vi "Create a Filter Bank from a Prototype Filter.vi"() -> ()   [LabVIEW 2023]
doc: "This example demonstrates how to use the <b>DFD Build Filter Bank from Prototype Filter</b> VI to create a cosine-modulated filter bank from prototype filter coefficients.\n\nComplete the following steps to use this VI:\n1) Run this VI.\n2) On the <b>Frequency Responses</b> tab, observe the magnitude and phase responses of the filter bank.\n3) On the <b>Distortions</b> tab, observe the aliasing, magnitude distortion, and phase distortion in the filter bank. The distortions are small.\n4) Change the value of <b>Band Counts</b>. \n5) Run this VI. Observe the <b>Distortions</b> tab. The distortions are large, which means this filter bank does not have perfect reconstruction. If you change <b>Band Counts</b>, you also must change the <b>Prototype Filter Coefficients</b>.\n6) To design a prototype filter, copy the coefficients to <b>Prototype Filter Coefficients</b> and set the proper value of <b>Band Counts</b>. Observe the frequency responses and distortions."
uses:
  <vilib>/addons/Digital Filter Design/_Objects.llb/DFD Phase Setting.ctl
  <vilib>/addons/Digital Filter Design/FilterBank.llb/FilterBankLib/DFD Build Filter Bank from Filter Coefficients.vi
  <vilib>/addons/Digital Filter Design/NI_DigFilter_FilterBank.lvlib
  <vilib>/addons/Digital Filter Design/NI_DigFilterLicensed.lvlib
panel:
  in  "Tab Control":enum32{"Frequency Responses", "Distortions"}(tab)
  out "Magnitude Responses":cluster{"Y":dbl[], "Y":dbl[]}[](graph)
  out "Phase Responses":cluster{"Y":dbl[], "Y":dbl[]}[](graph)
  out "Aliasing":cluster{dbl[], "values":dbl[]}(graph)
  out "Magnitude Distortion":cluster{dbl[], "values":dbl[]}(graph)
  out "Phase Distortion":cluster{dbl[], "values":dbl[]}(graph)
  in  "Band Counts":i32=4
  in  "Prototype Filter Coefficients":dbl[](array[numeric])=[3.82246474069644e-05, -0.0013784809253753554, 0.009144604896938757, 0.0003140814295197787, 0.00013518515431935828, 0.0003333316277785628, 0.0022112645736163537, -0.001110779285062549, -0.004449412805990734, -0.025388145079228278, -0.023860529399402756, -0.02350561463356747, -0.013170266328729315, 0.012862434811574027, 0.03883151987903549, 0.062049771616075604, 0.08864889782622157, 0.11056100576702955, 0.12668278199988298, 0.1370915002247963, 0.1370915002247963, 0.12668278199988298, 0.11056100576702955, 0.08864889782622157, 0.062049771616075604, 0.03883151987903549, 0.012862434811574027, -0.013170266328729315, -0.02350561463356747, -0.023860529399402756, -0.025388145079228278, -0.004449412805990734, -0.001110779285062549, 0.0022112645736163537, 0.0003333316277785628, 0.00013518515431935828, 0.0003140814295197787, 0.009144604896938757, -0.0013784809253753554, 3.82246474069644e-05]
  # "Select Help>>Show Context Help and move the cursor over the VI icon for more information."
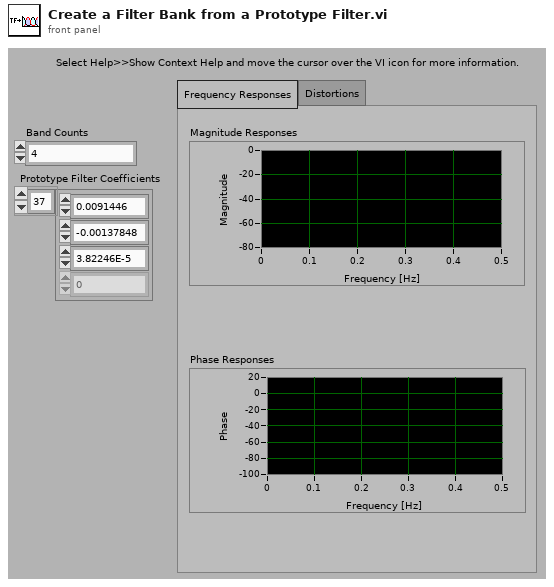
[diagram p1: front panel]
types:
  T1 = typedef "NI_DigFilterLicensed.lvlib/DFD Phase Setting.ctl" = cluster{"unwrap? (F)":bool, "degree? (F)":bool}
  T2 = typedef "NI_DigFilter_FilterBank.lvlib/DFD Filter Bank Obj.ctl" = cluster{"mFBank_AnalysisFilters":T3[], "mFBank_SynthesisFilters":T3[], "mFBank_#Bands":i32, "mFBank_ProcMethod":T8, "mFBank_Coeffs":dbl[], "mFBank_Gain":dbl, "mFBank_Delay":i32, "mFBank_Type":T9}
  T3 = typedef "NI_DigFilterLicensed.lvlib/DFD Multirate Filter Obj.ctl" = cluster{"mMRate_Structure":enum16{"CIC", "FIR", "IIR", "Lattice"}, "mMRate_Mode":T4, "mMRate_Factor":i32, "mMRate_FIRParams":cluster{"mMRate_FIR_H":dbl[], "mMRate_FIR_IsNyquist?":bool, "mMRate_FIR_IsSymmetric?":bool}, "mMRate_CICParams":cluster{"mMRate_CIC_#Stage":i32, "mMRate_CIC_Lag":i32, "mMRate_CIC_Type":enum16{"Lowpass", "Highpass"}}, "mMRate_Order":i32, "mMRate_Version":string, "mMRate_Comments":string, "mMRate_RationalFactor":cluster{"mMRate_L":i32, "mMRate_M":i32}, "mMRate_Fs":dbl, "mMRate_Quantized?":bool, "mMRate_QFilterGain":dbl, "mMRate_CoefWl":i16, "mMRate_Scaling":cluster{"mMRate_ScaleByPowerOf2?":bool, "mMRate_ScaleType":T5}, "mMRate_InputWl":i16, "mMRate_OutputWl":i16, "mMRate_OutputMode":T6, "mMRate_MultMode":T7, "mMRate_BitPruning":bool, "mMRate_GainWl":i16, "mMRate_OutputFwl":i16, "mMRate_SumIwl":i16, "mMRate_InputIwl ":i16, "mMRate_SumWl":i16, "mMRate_CoefIwl":i16}
  T4 = typedef "NI_DigFilterLicensed.lvlib/DFD Multirate Mode.ctl" = i16
  T5 = typedef "NI_DigFilterLicensed.lvlib/DFD Coef Norm Type.ctl" = enum16{"No Norm", "Time Domain 1-Norm", "Time Domain 2-Norm", "Time Domain Inf-Norm"}
  T6 = typedef "NI_DigFilterLicensed.lvlib/DFD Round-off Mode.ctl" = enum16{"Nearest", "Truncation"}
  T7 = typedef "NI_DigFilterLicensed.lvlib/DFD FXP MRate Multiply Mode.ctl" = enum16{"Truncated", "Full"}
  T8 = typedef "NI_DigFilter_FilterBank.lvlib/DFD Filter Bank Processing Method.ctl" = enum16{"General", "2-Band QMF Lattice", "Cosine-Modulated"}
  T9 = typedef "NI_DigFilter_FilterBank.lvlib/DFD Filter Bank Type.ctl" = u16
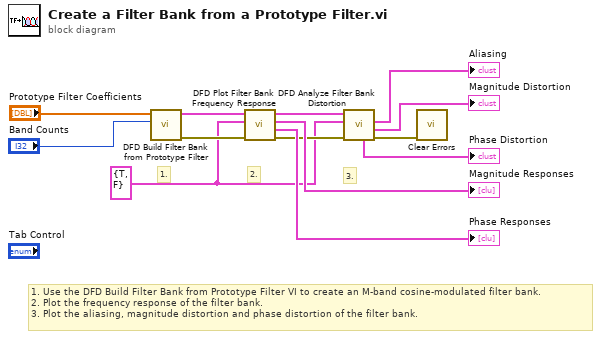
[diagram p0: block diagram]
diagram:
  w1 = T1 {"unwrap? (F)"=TRUE, "degree? (F)"=FALSE} ("Phase View")
  # "3."
  # "2."
  # "1."
  # "1. Use the DFD Build Filter Bank from Prototype Filter VI to create an M-band cosine-modulated filter bank.\n2. Plot the frequency response of the filter bank.\n3. Plot the aliasing, magnitude distortion and phase distortion of the filter bank."
  n1 = call-poly <vilib>:"DFD Build Filter Bank from Prototype Filter.vi"("band counts"="Band Counts", "h(n)"="Prototype Filter Coefficients") -> ("error out"=w10:errorcluster, "filter bank out"=w11:T2)  [unwired: 8 in]
  n2 = call <vilib>:"DFD Plot Filter Bank Frequency Response.vi"("error in (no error)"=w10, "phase view"=w1, "filter bank in"=w11) -> ("error out"=w6:errorcluster, "phase responses"=→"Phase Responses":cluster{"Y":dbl[], "Y":dbl[]}[], "magnitude responses"=→"Magnitude Responses":cluster{"Y":dbl[], "Y":dbl[]}[], "filter bank out"=w7:T2)  [unwired: 5 in]
  n3 = call <vilib>:"DFD Analyze Filter Bank Distortion.vi"("error in (no error)"=w6, "phase view"=w1, "filter bank in"=w7) -> ("error out"=w5:errorcluster, "magnitude distortion"=→"Magnitude Distortion":cluster{dbl[], "values":dbl[]}, "aliasing"=→"Aliasing":cluster{dbl[], "values":dbl[]}, "phase distortion"=→"Phase Distortion":cluster{dbl[], "values":dbl[]})  [unwired: 4 in, 1 out]
  n4 = call <vilib>:"Clear Errors.vi"("error in (no error)"=w5) -> ()  [unwired: 5 in, 2 out]
